vi "Unpack Value Change.vi"(11 "ValueChangeMsg In":refnum<class "ValueChangeMsg.lvclass">) -> (1 "New Value":variant, 2 "Time":u32, 3 "Name":string, 5 "Ctl Refnum":refnum<vi>)   [LabVIEW 2015, in "ActorEvents.lvlib" / "ValueChangeMsg.lvclass"]
doc: "<License>\nCopyright © 2017 Composed Systems, LLC | All rights reserved\nwww.composed.io\n\nAuthor: Ethan Stern <ethan.stern@composed.io>\n\nThis software is provided \"AS IS\" WITHOUT WARRANTIES, either express or implied, AND IS FOR EDUCATIONAL PURPOSES ONLY.\n</License>"
uses:
  ValueChangeMsg.lvclass
  ValueChangeMsg.lvclass/ValueChangeMsg.ctl
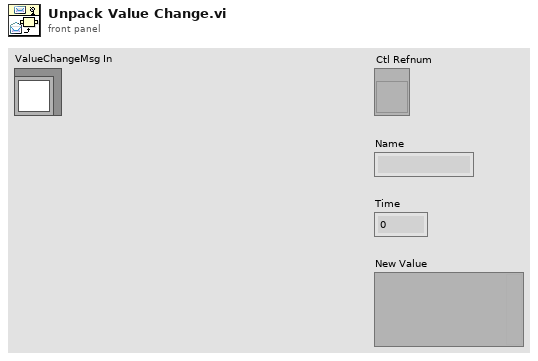
[diagram p1: front panel]
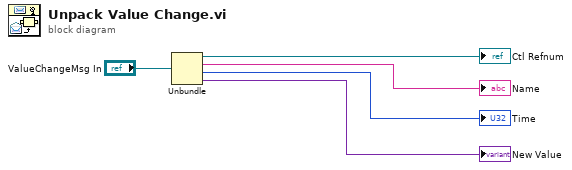
[diagram p0: block diagram]
diagram:
  n1 = Unbundle("ValueChangeMsg In") -> (→"Ctl Refnum":refnum<vi>, →"Name":string, →"Time":u32, →"New Value":variant)
